vi "Robot Global Data.vi"() -> ()   [LabVIEW 2012]
doc: "This global VI can contain as many global variables as you need. Place a control on the panel, give it a good name. To read or write to it from a VI, drag the icon to the diagram of that VI. You can also drag from the project. Click on the node to change which global you access. You shouldn't have multiple locations writing to a global or it will cause a race-condition."
uses:
  <vilib>/Rock Robotics/WPI/Camera/WPI_CameraImageSize.ctl
  <vilib>/Rock Robotics/WPI/DriverStation/WPI_DriverStationRobotMode2.ctl
panel:
  out "Tail Closed":bool
  in  "Climber Arm Inches Per Volt":dbl
  in  "Climber Arm Position":dbl
  in  "Drive Ramp Constant Y":dbl
  in  "Drive Mechanical Deadband Y":dbl
  in  "Drive Mechanical Deadband X":dbl
  in  "Drive Ramp Constant X":dbl
  in  "TARF Angle Offset":dbl=60.0
  in  "Deadband Scale Calc":dbl
  in  "Driver Deadband":dbl=0.2
  in  "Climber Counter Max":u8=19
  out "TARF At Desired Angle":bool
  in  "Manual TARF Control Rate":dbl=10.0
  in  "TARF Angle Tolerance":dbl=1.0
  in  "Desired TARF Angle":dbl
  in  "TARF Angle Right":dbl
  in  "TARF Angle Left":dbl
  in  "Robot Mode":T1
  in  "LED toggle rate (ms)":u32=20
  in  "image size":T2=enum."320x240"
  in  "Enable Vision":bool
  # "deg"
  # "Deg/Sec"
  # "Number of counts to\nreach the top of the tower"
  # "Rear limit switches reset encoder counter\ntherefore offset by the maximum TARF angle."
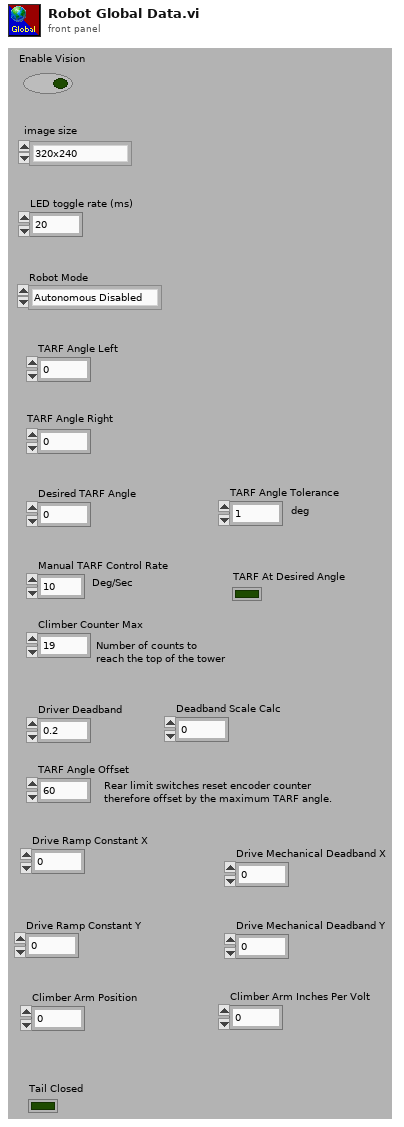
[diagram p1: front panel]
types:
  T1 = typedef "WPI_DriverStationRobotMode2.ctl" = enum16{"Autonomous Disabled", "Autonomous Enabled", "Teleop Disabled", "Teleop Enabled", "Timeout", "Finish", "Test Disabled", "Test Enabled"}
  T2 = typedef "WPI_CameraImageSize.ctl" = enum16{"640x480", "320x240", "160x120"}
diagram:
